vi "06TRM800.vi"() -> ()   [LabVIEW 2015]
panel:
  in  "INC 14 MPH 10":bool
  in  "INC 12 MPH 10":bool
  in  "INC 10 MPH 10":bool
  in  "INC 8 MPH 10":bool
  in  "INC 6 MPH 10":bool
  in  "INC 4 MPH 10":bool
  in  "INC 2 MPH 10":bool
  in  "INC 0 MPH 10":bool
  in  "INC 14 MPH 8":bool
  in  "INC 12 MPH 8":bool
  in  "INC 10 MPH 8":bool
  in  "INC 8 MPH 8":bool
  in  "INC 6 MPH 8":bool
  in  "INC 4 MPH 8":bool
  in  "INC 2 MPH 8":bool
  in  "INC 0 MPH 8":bool
  in  "INC 14 MPH 6":bool
  in  "INC 12 MPH 6":bool
  in  "INC 10 MPH 6":bool
  in  "INC 8 MPH 6":bool
  in  "INC 6 MPH 6":bool
  in  "INC 4 MPH 6":bool
  in  "INC 2 MPH 6":bool
  in  "INC 0 MPH 6":bool
  in  "INC 14 MPH 4":bool
  in  "INC 12 MPH 4":bool
  in  "INC 10 MPH 4":bool
  in  "INC 8 MPH 4":bool
  in  "INC 6 MPH 4":bool
  in  "INC 4 MPH 4":bool
  in  "INC 2 MPH 4":bool
  in  "INC 0 MPH 4":bool
  in  "INC 14 MPH 2":bool
  in  "INC 12 MPH 2":bool
  in  "INC 10 MPH 2":bool
  in  "INC 8 MPH 2":bool
  in  "INC 6 MPH 2":bool
  in  "INC 4 MPH 2":bool
  in  "INC 2 MPH 2":bool
  in  "INC 0 MPH 2":bool
  in  "INC 14 MPH 0":bool
  in  "INC 12 MPH 0":bool
  in  "INC 10 MPH 0":bool
  in  "INC 8 MPH 0":bool
  in  "INC 6 MPH 0":bool
  in  "INC 4 MPH 0":bool
  in  "INC 2 MPH 0":bool
  in  "INC 0 MPH 0":bool
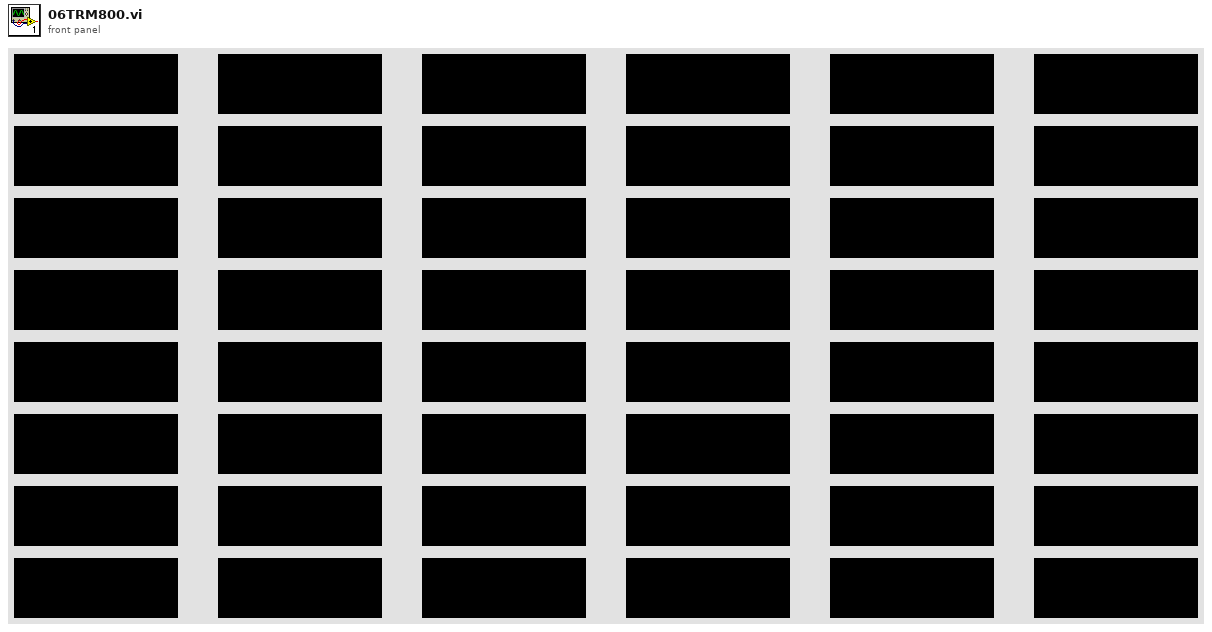
[diagram p1: front panel]
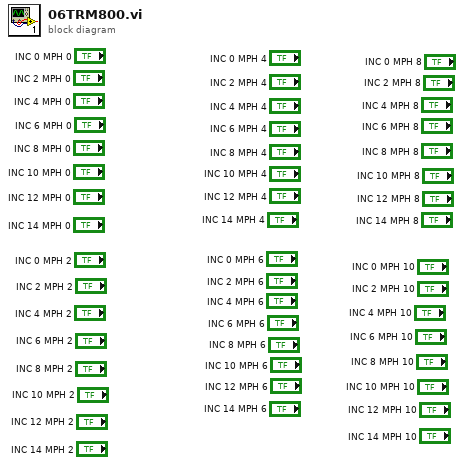
[diagram p0: block diagram]
diagram:
